vi "Get_Driver_Path.vi"(11 "Driver Filename":string) -> (3 "Driver Path":path)   [LabVIEW 2020, in "DriverCommon.lvlib"]
uses:
  DriverCommon.lvlib
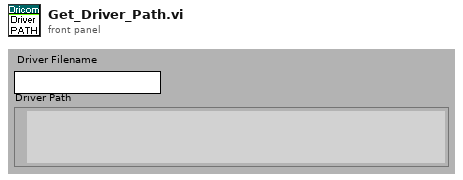
[diagram p1: front panel]
types:
  T1 = enum32{"invalid app kind", "Development System", "Run Time System", "Student Edition", "Embedded LabVIEW", "Evaluation", "Custom"}
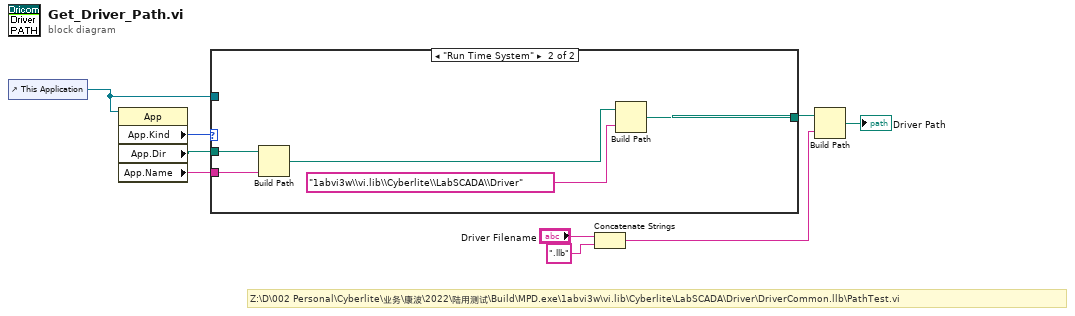
[diagram p0: block diagram]
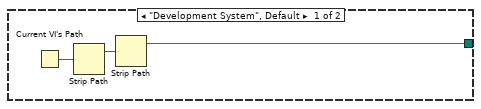
[diagram p2: hidden frame]
diagram:
  # "Z:\\D\\002 Personal\\Cyberlite\\业务\\康波\\2022\\陆用测试\\Build\\MPD.exe\\1abvi3w\\vi.lib\\Cyberlite\\LabSCADA\\Driver\\DriverCommon.llb\\PathTest.vi"
  n1 = control-ref of="This Application"() -> (w5:refnum<vi>)
  n2 = property class="App"(reference=w5) -> ("App.Kind"=w6:T1, "App.Dir"=w2:path, "App.Name"=w1:string)  [unwired: 1 in, 2 out]
  n3 = case shown="\"Run Time System\"" w6 {
    tunnel: w5 -> [_ _]
    tunnel: [w10 w16] -> w4
    tunnel: w2 -> [_ w15]
    tunnel: w1 -> [_ w14]
    frame "Development System", Default {
      n4 = Current VI's Path() -> (path=w11:path)
      n5 = Strip Path(path=w11) -> (stripped path=w12:path)  [unwired: 1 out]
      n6 = Strip Path(path=w12) -> (stripped path=w10:path)  [unwired: 1 out]
    }
    frame "Run Time System" {
      n7 = Build Path(base path=w15, name or relative path=w14) -> (appended path=w13:path)
      n8 = Build Path(base path=w13, name or relative path="1abvi3w\\vi.lib\\Cyberlite\\LabSCADA\\Driver") -> (appended path=w16:path)
    }
  }
  n9 = Concatenate Strings("Driver Filename", ".llb" ("string")) -> (w7:string)
  n10 = Build Path(base path=w4, name or relative path=w7) -> (appended path=→"Driver Path":path)
